vi "Read Daq ini.vi"(8 "error in":errorcluster) -> (0 "AI Channels":string[](array[string]), 1 "Max Voltage":T1[](array[typedef])=[enum."1 V", enum."1 V", enum."1 V", enum."1 V"], 2 "Device":u16(ring), 3 "Devices":string[](array[string]), 4 "samples per read":i32=10 min=1 max=25 step=1, 5 "DeviceName":string, 6 "Data rate (hz)":dbl=500.0 min=1.0 max=2500.0 step=1.0 format="%#.0f", 7 "AI voltage":dbl[](array[numeric]), 11 "Buffer":i32)   [LabVIEW 2015]
uses:
  AI voltages.ctl
  Calibration and Function folders.ctl
  DAQ configuration/Sensor buffer command.ctl
  <vilib>/Utility/config.llb/Read Key (Double).vi
  <vilib>/Utility/config.llb/Read Key (I32).vi
  <vilib>/Utility/config.llb/Read Key (String).vi
  <vilib>/Utility/config.llb/NI_LVConfig.lvlib
panel:
  out "error out":errorcluster
  in  "Max Voltage Default":T1=enum."1 V"
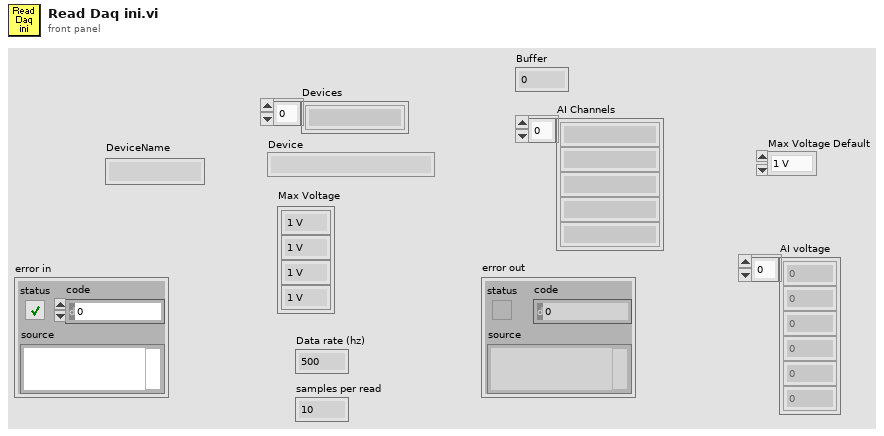
[diagram p1: front panel]
types:
  T1 = typedef "AI voltages.ctl" = enum16{"20 V", "10 V", "5 V", "4 V", "2.5 V", "2 V", "1.25 V", "1 V"}
  T2 = typedef "Sensor buffer command.ctl" = enum16{"read average", "read recent", "read all", "write", "set buffer size", "Read channel config", "Write channel config", "clear"}
  T3 = typedef "Calibration and Function folders.ctl" = enum16{"Sensors", "Functions", "Config File", "PublicAppFolder", "New ini File", "Set Config File", "Delete ini File"}
  T4 = typedef "NI_LVConfig.lvlib/Config Data RefNum.ctl" = refnum<k1>
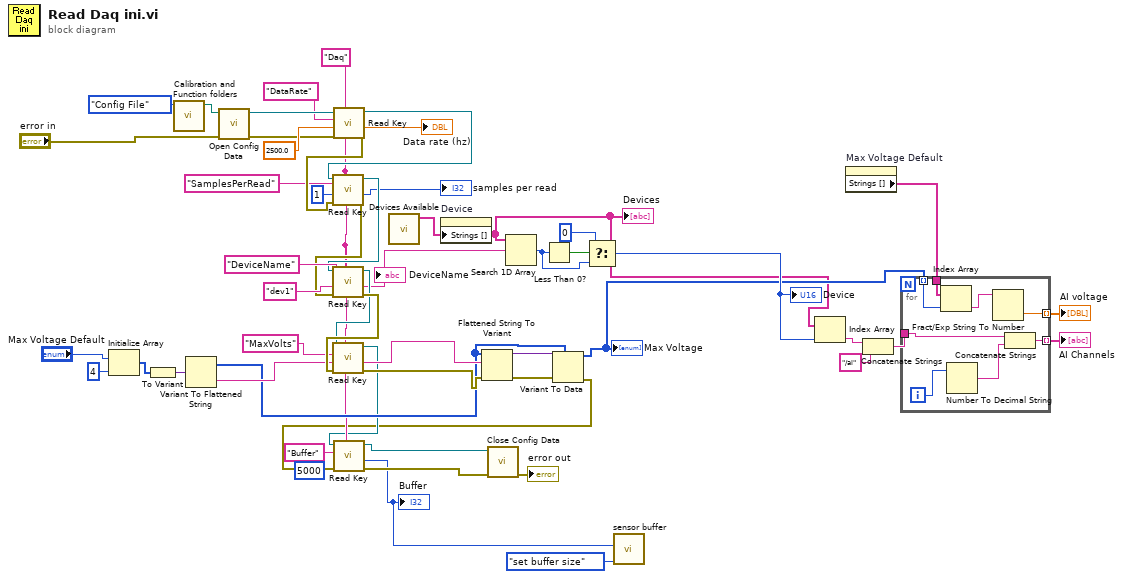
[diagram p0: block diagram]
diagram:
  w13 = "Daq" ("section")
  n1 = Initialize Array("Max Voltage Default", 4 ("dimension size")) -> (w28:T1[])
  n2 = To Variant(anything=w28) -> (Variant=w38:variant)
  n3 = call "Calibration and Function folders.vi"("Folder"=Calibration_and_Function_folders."Config File") -> ("Selected Folder"=w1:path)  [unwired: 9 in, 1 out]
  n4 = Variant To Flattened String(Variant=w38) -> (data string=w37:string, 1:w31:i16[])
  n5 = call <vilib>:"Open Config Data.vi"("error in (no error)"="error in", "configuration file path"=w1) -> ("error out"=w47:errorcluster, "refnum"=w53:T4)  [unwired: 7 in, 1 out]
  n6 = call-poly <vilib>:"Read Key.vi"("section"=w13, "error in (no error)"=w47, "default value"=2500.0, "key"="DataRate", "refnum"=w53) -> ("error out"=w48:errorcluster, "value"=→"Data rate (hz)":dbl, "refnum out"=w49:T4)  [unwired: 3 in, 1 out]
  n7 = call-poly <vilib>:"Read Key.vi"("section"=w13, "error in (no error)"=w48, "default value"=1, "key"="SamplesPerRead", "refnum"=w49) -> ("error out"=w43:errorcluster, "value"=→"samples per read":i32, "refnum out"=w42:T4)  [unwired: 3 in, 1 out]
  n8 = call-poly <vilib>:"Read Key.vi"("section"=w13, "error in (no error)"=w43, "default value"="dev1", "key"="DeviceName", "refnum"=w42) -> ("error out"=w40:errorcluster, "value"=w3:string, "refnum out"=w36:T4)  [unwired: 3 in, 1 out]
  "DeviceName" <- w3
  n9 = call-poly <vilib>:"Read Key.vi"("section"=w13, "error in (no error)"=w40, "default value"=w37, "key"="MaxVolts", "refnum"=w36) -> ("error out"=w32:errorcluster, "value"=w35:string, "refnum out"=w12:T4)  [unwired: 3 in, 1 out]
  n10 = call "Devices Available.vi"() -> ("Devices"=w4:string[])  [unwired: 7 in, 4 out]
  "Devices" <- w4
  n11 = property on="Device" class="Ring (strict)"("Strings []"=w4) -> ()  [unwired: 2 in, 2 out]
  n12 = Flattened String To Variant(4:w32, 6:w35, 7:w31) -> (0:w33:errorcluster, 3:w34:variant)
  n13 = Search 1D Array(1D array=w4, element=w3) -> (index of element=w26:i32)  [unwired: 1 in]
  n14 = Less Than 0?(x=w26) -> (x < 0?=w27:bool)
  n15 = Variant To Data(error in=w33, type=w31, Variant=w34) -> (data=w17:i16[], error out=w10:errorcluster)
  "Max Voltage" <- w17
  n16 = call-poly <vilib>:"Read Key.vi"("section"=w13, "error in (no error)"=w10, "default value"=5000, "key"="Buffer", "refnum"=w12) -> ("error out"=w7:errorcluster, "value"=w5:i32, "refnum out"=w11:T4)  [unwired: 3 in, 1 out]
  "Buffer" <- w5
  n17 = call <vilib>:"Close Config Data.vi"("error in (no error)"=w7, "refnum"=w11) -> ("error out"=→"error out":errorcluster)  [unwired: 8 in, 1 out]
  n18 = Select(t=0, s=w27, f=w26) -> (s? t:f=w18:i32)
  "Device" <- w18
  n19 = call "sensor buffer.vi"("command"=Sensor_buffer_command."set buffer size", "max array size"=w5) -> ()  [unwired: 5 in, 5 out]
  n20 = Index Array(array=w4, index=w18) -> (element=w21:string)
  n21 = property on="Max Voltage Default" class="Enum (strict)"() -> ("Strings []"=w14:string[])  [unwired: 2 in, 2 out]
  n22 = Concatenate Strings(w21, "/ai") -> (w19:string)
  n23 = for {
    tunnel: w19 -> [w61]
    tunnel: [w58] -> w15 mode=indexing
    tunnel: w14 -> [w57]
    tunnel: w17 -> [w56] mode=indexing
    tunnel: [w54] -> w16 mode=indexing
    i -> [w60]
    n24 = Index Array(array=w57, index=w56) -> (element=w55:string)
    n25 = Number To Decimal String(number=w60) -> (decimal integer string=w59:string)  [unwired: 1 in]
    n26 = Fract/Exp String To Number(string=w55) -> (number=w54:dbl)  [unwired: 3 in, 1 out]
    n27 = Concatenate Strings(w61, w59) -> (w58:string)
  }
  "AI voltage" <- w16
  "AI Channels" <- w15
